vi "Main.vi"(10 "MCP Sub Panel":refnum<vi>, 11 "Module Admin":refnum<class "Delacor_lib_QMH_Module Admin.lvclass">) -> ()   [LabVIEW 2020, in "Money Control Pane.lvlib"]
doc: "This template is based off of the Queued Message Handler design pattern and the Queued Message Handler project template that ships with LabVIEW.\n\nThe main difference is that the queue is private to this module and communication between modules is performed via Broadcast and Request events.\n\nRequest events are wrapped in public API methods and are handled in the Event Handling Loop (EHL) of this VI. Any module can register for Broadcast events sent by this module. The EHL generates messages based on user interface actions.\n\nThe Message Handling Loop (MHL) processes messages generated by the EHL, or by other messages. The messages are string values, so new messages can be added easily to the Message Cases case structure in the MHL. Each message cluster can also provide an optional value for Message Data, which is a variant that can be converted to whatever message-specific data is required.\n_____\nBased on Delacor QMH Project Template 5.0.0.82."
uses:
  Money Control Pane.lvlib
  <vilib>/Delacor/Delacor QMH/Libraries/Module Admin_class/Delacor_lib_QMH_Module Admin.lvclass
  Module Data--cluster.ctl
  Stop Argument--cluster.ctl
  <vilib>/Delacor/Delacor QMH/Libraries/Message Queue_class/Delacor_lib_QMH_Message Queue.lvclass/Delacor_lib_QMH_Message Queue.ctl
  <vilib>/Delacor/Delacor QMH/Libraries/Module Admin_class/Delacor_lib_QMH_Module Admin.lvclass/Delacor_lib_QMH_Module Admin.ctl
  Configuration Change Argument--cluster.ctl
  TypeDefinitions/CurrencyEnum.ctl
  <vilib>/Utility/miscctls.llb/LVPointTypeDef.ctl
  <vilib>/Delacor/Delacor QMH/Libraries/Message Queue_class/Delacor_lib_QMH_Enqueue Message (Single).vi
  <vilib>/Delacor/Delacor QMH/Libraries/Module Admin_class/Delacor_lib_QMH_Get External Launch.vi
  <vilib>/Utility/error.llb/Error Cluster From Error Code.vi
  <vilib>/ErrorRing/Error Ring.xnode
  <vilib>/Delacor/Delacor QMH/Libraries/Message Queue_class/Delacor_lib_QMH_Message Queue.lvclass
  Config Files Management/Config File Management.lvlib
panel:
  out "value":dbl
  in  "Coins":T1
  out "error out":errorcluster
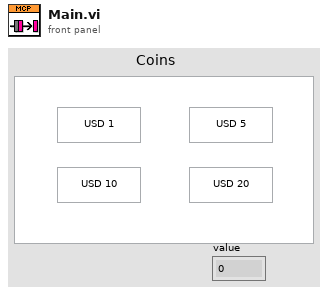
[diagram p1: front panel]
types:
  T1 = cluster{"Coin 1":bool, "Coin 2":bool, "Coin 3":bool, "Coin 4":bool}
  T2 = typedef "Money Control Pane.lvlib/Request Events--cluster.ctl" = cluster{"Stop Module":refnum<user-event>, "Show Panel":refnum<user-event>, "Hide Panel":refnum<user-event>, "Get Module Execution Status":refnum<user-event>, "Show Diagram":refnum<user-event>, "Configuration Change":refnum<user-event>}
  T3 = typedef "Money Control Pane.lvlib/Module Data--cluster.ctl" = cluster{"Status":string, "Coin Array":string[], "Values":dbl[]}
  T4 = enum32{"invalid lock state", "Not Locked", "Locked (No Password)", "Password-protected"}
  T5 = typedef "Money Control Pane.lvlib/Stop Argument--cluster.ctl" = cluster{"Origin":string, "Exit via Stop Module Req?":bool, "Wait for Module to stop?":bool}
  T6 = typedef "Money Control Pane.lvlib/Configuration Change Argument--cluster.ctl" = cluster{"Enum":T7}
  T7 = typedef "CurrencyEnum.ctl" = enum16{"USD", "MXN", "EUR", "GBP"}
  T8 = typedef "LVPointTypeDef.ctl" = cluster{"Horizontal":i16, "Vertical":i16}
  T9 = enum32{"Invalid", "Standard", "Closed", "Hidden", "Minimized", "Maximized"}
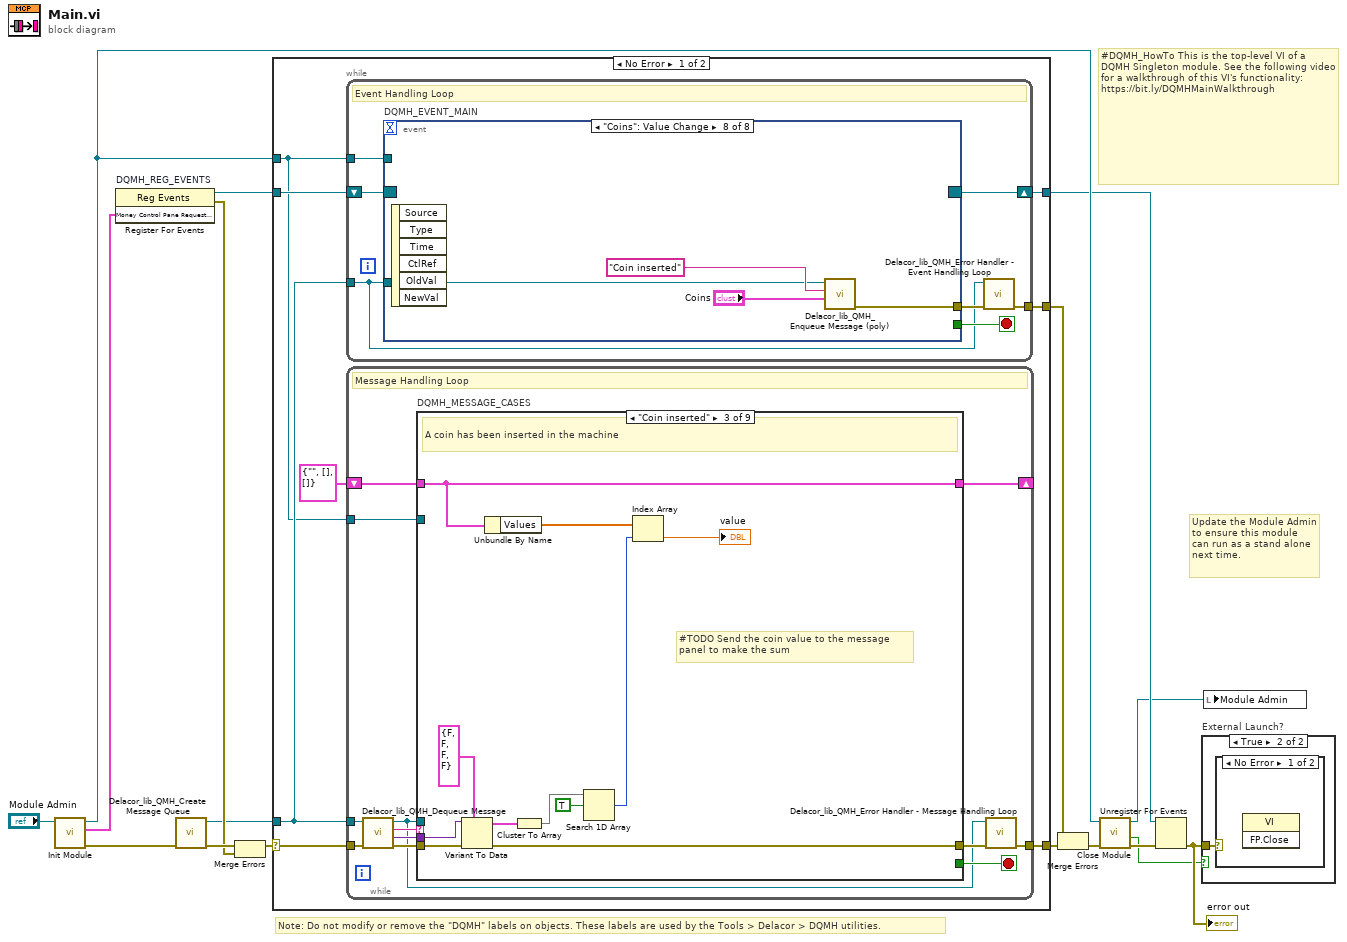
[diagram p0: block diagram]
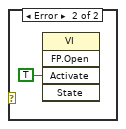
[diagram p3: hidden frame]
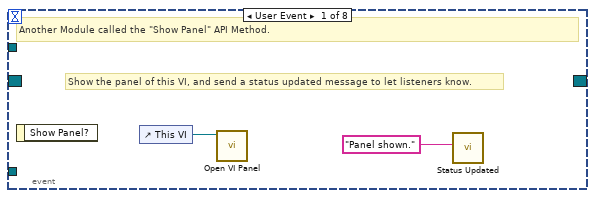
[diagram p4: hidden frame]
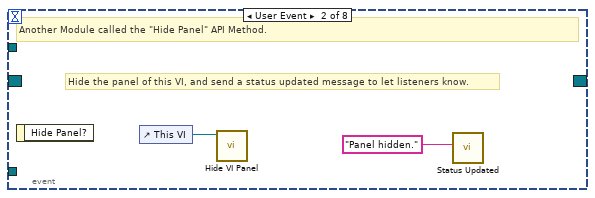
[diagram p5: hidden frame]
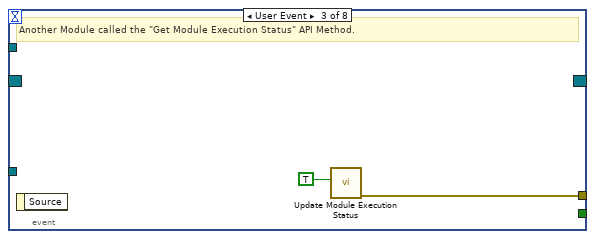
[diagram p6: hidden frame]
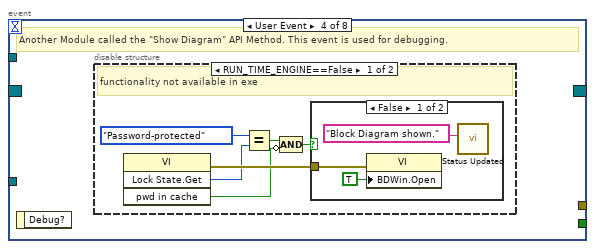
[diagram p7: hidden frame]
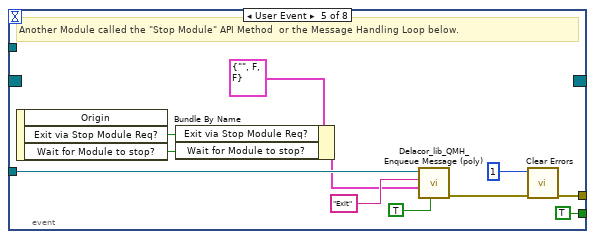
[diagram p10: hidden frame]
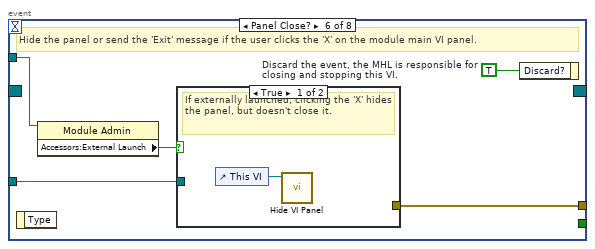
[diagram p11: hidden frame]
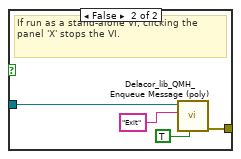
[diagram p12: hidden frame]
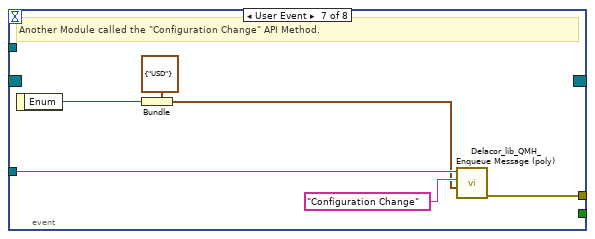
[diagram p13: hidden frame]
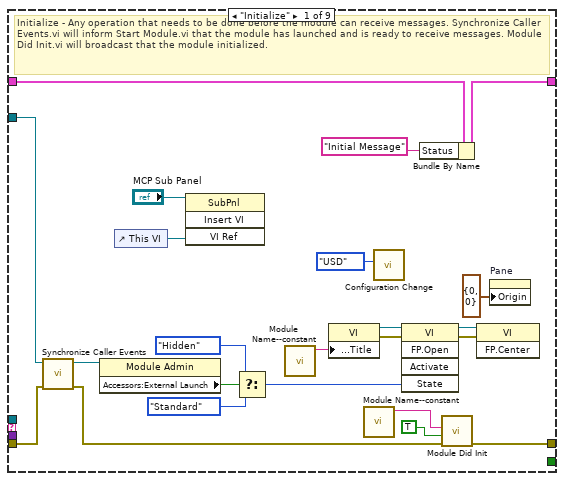
[diagram p14: hidden frame]
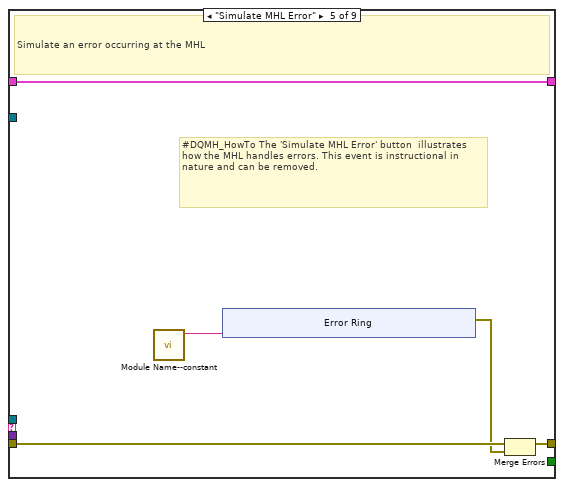
[diagram p17: hidden frame]
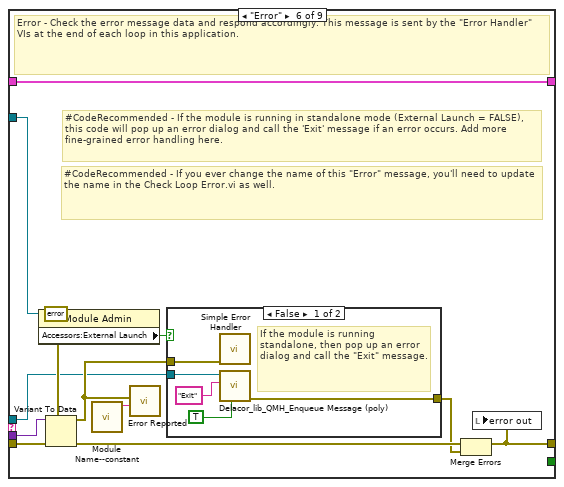
[diagram p18: hidden frame]
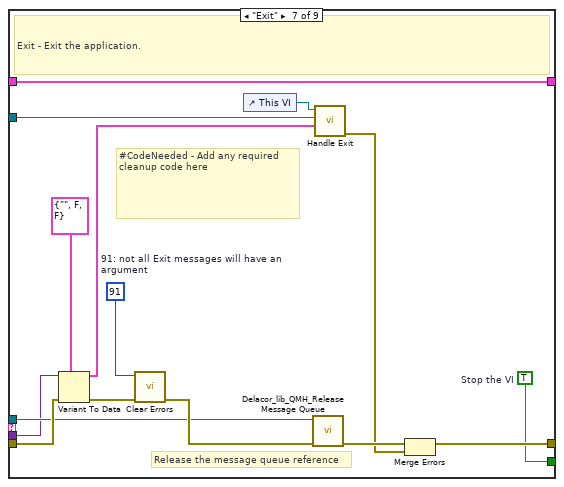
[diagram p20: hidden frame]
diagram:
  # "#DQMH_HowTo This is the top-level VI of a DQMH Singleton module. See the following video for a walkthrough of this VI's functionality: https://bit.ly/DQMHMainWalkthrough"
  # "Note: Do not modify or remove the \"DQMH\" labels on objects. These labels are used by the Tools > Delacor > DQMH utilities."
  # "Update the Module Admin to ensure this module can run as a stand alone next time."
  n1 = call "Init Module.vi"("Singleton Module Admin in"="Module Admin") -> ("error out"=w16:errorcluster, "Money Control Pane Request Events"=w5:T2, "Singleton Module Admin out"=w8:refnum<class "Delacor_lib_QMH_Module Admin.lvclass">)  [unwired: 8 in]
  n2 = register-events "DQMH_REG_EVENTS"(w5) -> (reference out=w6:refnum<event-registration>, error out=w9:errorcluster)  [unwired: 2 in]
  n3 = call <vilib>:"Delacor_lib_QMH_Create Message Queue.vi"("error in (no error)"=w16) -> ("error out"=w11:errorcluster, "Message Queue"=w4:refnum<class "Delacor_lib_QMH_Message Queue.lvclass">)  [unwired: 9 in]
  n4 = Merge Errors(w11, w9) -> (w10:errorcluster)
  n5 = case shown="No Error" w10 {
    selector: w10 -> [w23 w204]
    tunnel: [w25 w203] -> w17
    tunnel: [w22 w209] -> w7
    tunnel: w6 -> [w20 w209]
    tunnel: w4 -> [w19 w202]
    tunnel: [w24 _] -> w14
    tunnel: w8 -> [w18 w205]
    frame No Error {
      n6 = while {
        tunnel: w19 -> [w26]
        shift-right: [w29] -> w22
        shift-left: w20 -> [w30]
        tunnel: [w31] -> w24
        tunnel: w18 -> [w27]
        stop <- w28 stop-if-true
        # "Event Handling Loop"
        n7 = event "DQMH_EVENT_MAIN" shown="[7] \"Coins\": Value Change" {
          selector: w30 -> [_ _ _ _ _ _ _ _]
          dyn-events: [_ _ _ _ _ _ _ _] -> w29
          timeout: _ -> [_ _ _ _ _ _ _ _]
          tunnel: [_ _ _ _ TRUE ("Discard?") _ _ _] -> w28
          tunnel: w26 -> [_ _ _ _ w54 w61 w74 w77]
          tunnel: [_ _ w38 _ w57 w63 w69 w76] -> w32
          tunnel: w27 -> [_ _ _ _ _ w60 _ _]
          event User Event {
            # "Show the panel of this VI, and send a status updated message to let listeners know."
            # "Another Module called the \"Show Panel\" API Method."
            n8 = event-data() -> ()  [unwired: 1 in, 1 out]
            n9 = control-ref of="This VI"() -> (w34:refnum<vi>)
            n10 = call "Open VI Panel.vi"("VI"=w34) -> ()  [unwired: 10 in, 1 out]
            n11 = call "Status Updated.vi"("Status"="Panel shown." ("format string")) -> ()  [unwired: 10 in, 1 out]
          }
          event User Event {
            # "Hide the panel of this VI, and send a status updated message to let listeners know."
            # "Another Module called the \"Hide Panel\" API Method."
            n12 = event-data() -> ()  [unwired: 1 in, 1 out]
            n13 = control-ref of="This VI"() -> (w36:refnum<vi>)
            n14 = call "Hide VI Panel.vi"("VI"=w36) -> ()  [unwired: 10 in, 1 out]
            n15 = call "Status Updated.vi"("Status"="Panel hidden." ("format string")) -> ()  [unwired: 10 in, 1 out]
          }
          event User Event {
            # "Another Module called the \"Get Module Execution Status\" API Method."
            n16 = event-data() -> ()  [unwired: 1 in, 1 out]
            n17 = call "Update Module Execution Status.vi"("Running?"=TRUE) -> ("error out"=w38:errorcluster)  [unwired: 10 in]
          }
          event User Event {
            # "Another Module called the \"Show Diagram\" API Method. This event is used for debugging."
            n18 = event-data() -> ()  [unwired: 1 in, 1 out]
            n19 = disable-structure shown="RUN_TIME_ENGINE==False" {
              frame condition #0 (active) {
                # "functionality not available in exe"
                n20 = invoke class="VI" method="Lock State.Get"() -> (error out=w44:errorcluster, "Get Lock State"=w43:T4, "pwd in cache"=w40:bool)  [unwired: 4 in, 1 out]
                n21 = Equal?(x=T4."Password-protected", y=w43) -> (x = y?=w41:bool)
                n22 = Compound Arithmetic op=AND(w41, invert w40) -> (w39:bool)
                n23 = case shown="False" w39 {
                  tunnel: w44 -> [w47 _]
                  frame False {
                    n24 = property class="VI"(error in=w47, "BDWin.Open"=TRUE ("Block Diagram Window:Open")) -> ()  [unwired: 1 in, 2 out]
                    n25 = call "Status Updated.vi"("Status"="Block Diagram shown." ("format string")) -> ()  [unwired: 10 in, 1 out]
                  }
                  frame True {
                    # "Password-protected VI, and the password is not in the cache. Do not show the diagram."
                  }
                }
              }
              frame condition #1 {
              }
            }
          }
          event User Event {
            # "Another Module called the \"Stop Module\" API Method  or the Message Handling Loop below."
            n26 = event-data() -> ("Exit via Stop Module Req?"=w50:bool, "Wait for Module to stop?"=w49:bool)  [unwired: 1 in, 1 out]
            n27 = Bundle By Name(cluster=T5 {"Origin"="", "Exit via Stop Module Req?"=FALSE, "Wait for Module to stop?"=FALSE} ("Stop Argument"), "Exit via Stop Module Req?"=w50, "Wait for Module to stop?"=w49) -> (w48:T5)
            n28 = call-poly <vilib>:"Delacor_lib_QMH_Enqueue Message (poly).vi"("Priority Message? (F)"=TRUE, "Message Data"=w48, "Message"="Exit", "Message Queue in"=w54) -> ("error out"=w58:errorcluster)  [unwired: 6 in, 1 out]
            n29 = call <vilib>:"Clear Errors.vi"("error in (no error)"=w58, "specific error code to clear (0: all)"=1) -> ("error out"=w57:errorcluster)  [unwired: 4 in, 1 out]
          }
          event Panel Close? {
            w62 = TRUE  # Discard the event, the MHL is responsible for closing and stopping this VI.
            # "Hide the panel or send the 'Exit' message if the user clicks the 'X' on the module main VI panel."
            n30 = event-data() -> ()  [unwired: 1 in, 1 out]
            n31 = property class="Module Admin"(reference=w60) -> ("Accessors:External Launch"=w59:bool)  [unwired: 1 in, 2 out]
            n32 = case shown="True" w59 {
              tunnel: w61 -> [_ w67]
              tunnel: [_ w68] -> w63
              frame True {
                # "If externally launched, clicking the 'X' hides the panel, but doesn't close it."
                n33 = control-ref of="This VI"() -> (w64:refnum<vi>)
                n34 = call "Hide VI Panel.vi"("VI"=w64) -> ()  [unwired: 10 in, 1 out]
              }
              frame False {
                # "If run as a stand-alone VI, clicking the panel 'X' stops the VI."
                n35 = call-poly <vilib>:"Delacor_lib_QMH_Enqueue Message (poly).vi"("Priority Message? (F)"=TRUE, "Message"="Exit", "Message Queue in"=w67) -> ("error out"=w68:errorcluster)  [unwired: 7 in, 1 out]
              }
            }
            n36 = event-data("Discard?"=w62) -> ()  [unwired: 1 in, 1 out]
          }
          event User Event {
            # "Another Module called the \"Configuration Change\" API Method."
            n37 = event-data() -> ("Enum"=w70:T7)  [unwired: 1 in]
            n38 = Bundle(cluster=T6 {"Enum"=enum."USD"} ("Configuration Change Argument"), "Enum"=w70) -> (w71:T6)
            n39 = call-poly <vilib>:"Delacor_lib_QMH_Enqueue Message (poly).vi"("Message Data"=w71, "Message"="Configuration Change", "Message Queue in"=w74) -> ("error out"=w69:errorcluster)  [unwired: 7 in, 1 out]
          }
          event "Coins": Value Change {
            n40 = event-data() -> ()  [unwired: 1 in, 6 out]
            n41 = call-poly <vilib>:"Delacor_lib_QMH_Enqueue Message (poly).vi"("Message Data"="Coins", "Message"="Coin inserted", "Message Queue in"=w77) -> ("error out"=w76:errorcluster)  [unwired: 7 in, 1 out]
          }
        }
        n42 = call-dynamic "Delacor_lib_QMH_Error Handler - Event Handling Loop.vi"("error in (no error)"=w32, "Message Queue in"=w26) -> ("dup error in"=w31:errorcluster)  [unwired: 8 in, 1 out]
      }
      n43 = while {
        tunnel: w19 -> [w81]
        shift-right: [w85] -> _
        shift-left: T3 {"Status"="", "Coin Array"=[], "Values"=[]} ("Data Cluster") -> [w86]
        tunnel: w23 -> [w89]
        tunnel: [w87] -> w25
        tunnel: w18 -> [w79]
        stop <- w84 stop-if-true
        # "Message Handling Loop"
        n44 = call-dynamic "Delacor_lib_QMH_Dequeue Message.vi"("error in (no error)"=w89, "Message Queue in"=w81) -> ("error out"=w88:errorcluster, "Message Data"=w82:variant, "Message"=w83:string, "Message Queue out"=w80:refnum<class "Delacor_lib_QMH_Message Queue.lvclass">)  [unwired: 6 in]
        n45 = case "DQMH_MESSAGE_CASES" shown="\"Coin inserted\"" w83 {
          selector: w83 -> [_ _ _ _ _ _ _ w174 _]
          tunnel: w80 -> [_ _ _ _ _ w144 w166 _ _]
          tunnel: w88 -> [w111 w115 w126 w128 w133 w151 w172 w176 w201]
          tunnel: [w109 w115 w125 w128 w132 w147 w169 w177 w188] -> w90
          tunnel: w86 -> [w100 w114 w119 w127 w130 w146 w165 w175 w200]
          tunnel: [w99 w114 w119 w127 w130 w146 w165 w175 w191] -> w85
          tunnel: [_ _ _ _ _ _ w164 _ _] -> w84
          tunnel: w82 -> [_ _ w124 _ _ w145 w163 _ w198]
          tunnel: w79 -> [w101 _ _ _ _ w143 w158 _ _]
          frame "Initialize" {
            # "Initialize - Any operation that needs to be done before the module can receive messages. Synchronize Caller Events.vi will inform Start Module.vi that the module has launched and is ready to receive messages. Module Did Init.vi will broadcast that the module initialized."
            n46 = call "Synchronize Caller Events.vi"("error in (no error)"=w111, "Singleton Module Admin in"=w101) -> ("error out"=w110:errorcluster, "Singleton Module Admin out"=w96:refnum<class "Delacor_lib_QMH_Module Admin.lvclass">)  [unwired: 8 in]
            n47 = property class="Module Admin"(reference=w96) -> ("Accessors:External Launch"=w105:bool)  [unwired: 1 in, 2 out]
            n48 = control-ref of="This VI"() -> (w92:refnum<vi>)
            n49 = invoke class="SubPnl" method="Insert VI"(reference="MCP Sub Panel", "VI Ref"=w92) -> ()  [unwired: 2 in, 4 out]
            n50 = Select(t=T9."Hidden" ("State"), s=w105, f=T9."Standard" ("State")) -> (s? t:f=w102:T9)
            n51 = call "Module Name--constant.vi"() -> ("Module Name"=w108:string)  [unwired: 11 in]
            n52 = property class="VI"("Front Panel.Title"=w108) -> (reference out=w107:refnum<vi>, error out=w113:errorcluster)  [unwired: 2 in]
            n53 = call "Module Name--constant.vi"() -> ("Module Name"=w97:string)  [unwired: 11 in]
            n54 = call "Configuration Change.vi"("Enum"=CurrencyEnum."USD") -> ()  [unwired: 10 in, 1 out]
            n55 = invoke class="VI" method="FP.Open"(reference=w107, error in=w113, "State"=w102) -> (reference out=w106:refnum<vi>, error out=w112:errorcluster)  [unwired: 2 in, 3 out]
            n56 = Bundle By Name(cluster=w100, "Status"="Initial Message" ("Initial Message")) -> (w99:T3)
            n57 = call "Module Did Init.vi"("error in (no error)"=w110, "Initialized?"=TRUE, "Origin"=w97) -> ("error out"=w109:errorcluster)  [unwired: 8 in]
            n58 = invoke class="VI" method="FP.Center"(reference=w106, error in=w112) -> ()  [unwired: 1 in, 3 out]
            n59 = property on="Pane" class="Pane"("Origin"=T8 {"Horizontal"=0, "Vertical"=0}) -> ()  [unwired: 2 in, 2 out]
          }
          frame "--- Module Specific ---" {
            # "Separator -- The following cases handle messages specific to this Module."
          }
          frame "Coin inserted" {
            # "#TODO Send the coin value to the message \npanel to make the sum"
            # "A coin has been inserted in the machine"
            n60 = Variant To Data(error in=w126, type=T1 {"Coin 1"=FALSE, "Coin 2"=FALSE, "Coin 3"=FALSE, "Coin 4"=FALSE} ("Coins"), Variant=w124) -> (data=w122:T1, error out=w125:errorcluster)
            n61 = Unbundle By Name(w119) -> ("Values"=w118:dbl[])
            n62 = Cluster To Array(cluster=w122) -> (array=w121:bool[])
            n63 = Search 1D Array(1D array=w121, element=TRUE) -> (index of element=w117:i32)  [unwired: 1 in]
            n64 = Index Array(array=w118, index=w117) -> (element=→"value":dbl)
          }
          frame "--- Exit and Error Handling---" {
            # "Separator - The following cases handle errors and exit messages."
          }
          frame "Simulate MHL Error" {
            # "#DQMH_HowTo The 'Simulate MHL Error' button  illustrates how the MHL handles errors. This event is instructional in nature and can be removed."
            # "Simulate an error occurring at the MHL"
            n65 = call "Module Name--constant.vi"() -> ("Module Name"=w129:string)  [unwired: 11 in]
            n66 = xnode "Error Ring"("parameter 0"=w129) -> ("error out"=w131:errorcluster)
            n67 = Merge Errors(w133, w131) -> (w132:errorcluster)
          }
          frame "Error" {
            # "#CodeRecommended - If you ever change the name of this \"Error\" message, you'll need to update the name in the Check Loop Error.vi as well."
            # "#CodeRecommended - If the module is running in standalone mode (External Launch = FALSE), this code will pop up an error dialog and call the 'Exit' message if an error occurs. Add more fine-grained error handling here."
            # "Error - Check the error message data and respond accordingly. This message is sent by the \"Error Handler\" VIs at the end of each loop in this application."
            n68 = property class="Module Admin"(reference=w143) -> ("Accessors:External Launch"=w142:bool)  [unwired: 1 in, 2 out]
            n69 = Variant To Data(error in=w151, type=errorcluster {"status"=FALSE, "code"=0, "source"=""} ("error constant"), Variant=w145) -> (data=w152:errorcluster, error out=w149:errorcluster)
            n70 = call "Module Name--constant.vi"() -> ("Module Name"=w141:string)  [unwired: 11 in]
            n71 = call "Error Reported.vi"("Additional Information"=w141, "Error"=w152) -> ()  [unwired: 9 in, 1 out]
            n72 = case shown="False" w142 {
              tunnel: [w157 _] -> w148
              tunnel: w144 -> [w155 _]
              tunnel: w152 -> [w156 _]
              frame False {
                # "If the module is running standalone, then pop up an error dialog and call the \"Exit\" message."
                n73 = call <vilib>:"Simple Error Handler.vi"("error in (no error)"=w156) -> ()  [unwired: 4 in, 5 out]
                n74 = call-poly <vilib>:"Delacor_lib_QMH_Enqueue Message (poly).vi"("Priority Message? (F)"=TRUE, "Message"="Exit", "Message Queue in"=w155) -> ("error out"=w157:errorcluster)  [unwired: 7 in, 1 out]
              }
              frame True {
                # "If the module was launched externally, calling the Error Reported broadcast VI is the only action performed by the \"Error\" message. The module's caller can then process the error appropriately."
              }
            }
            n75 = Merge Errors(w149, w148) -> (w147:errorcluster)
            n76 = local write "error out"(w147) -> ()
          }
          frame "Exit" {
            w162 = 91  # 91: not all Exit messages will have an argument
            w164 = TRUE  # Stop the VI
            # "Release the message queue reference"
            # "#CodeNeeded - Add any required cleanup code here"
            # "Exit - Exit the application."
            n77 = Variant To Data(error in=w172, type=T5 {"Origin"="", "Exit via Stop Module Req?"=FALSE, "Wait for Module to stop?"=FALSE} ("Stop Argument"), Variant=w163) -> (data=w160:T5, error out=w168:errorcluster)
            n78 = call <vilib>:"Clear Errors.vi"("error in (no error)"=w168, "specific error code to clear (0: all)"=w162) -> ("error out"=w171:errorcluster)  [unwired: 4 in, 1 out]
            n79 = control-ref of="This VI"() -> (w159:refnum<vi>)
            n80 = call-dynamic "Delacor_lib_QMH_Release Message Queue.vi"("error in (no error)"=w171, "Message Queue"=w166) -> ("error out"=w170:errorcluster)  [unwired: 9 in]
            n81 = call "Handle Exit.vi"("Stop Argument"=w160, "Admin in"=w158, "VI reference"=w159) -> ("error out"=w167:errorcluster)  [unwired: 7 in, 1 out]
            n82 = Merge Errors(w170, w167) -> (w169:errorcluster)
          }
          frame Default {
            # "'Default' case only runs if there is a message that isn't defined in any of the other cases.  Output a programming error."
            n83 = call "Module Name--constant.vi"() -> ("Module Name"=w173:string)  [unwired: 11 in]
            n84 = xnode "Error Ring"("parameter 0"=w174, "parameter 1"=w173) -> ("error out"=w178:errorcluster)
            n85 = Merge Errors(w176, w178) -> (w177:errorcluster)
          }
          frame "Configuration Change" {
            # "Sets a configuration change done by the settings window or the VI itself."
            n86 = Variant To Data(error in=w201, type=T6 {"Enum"=enum."USD"} ("Configuration Change Argument"), Variant=w198) -> (error out=w199:errorcluster)  [unwired: 1 out]
            n87 = call "Create Currency Map.vi"() -> ("error out"=w187:errorcluster, "Value"=w190:dbl[], "Denomination"=w189:string[])  [unwired: 9 in]
            n88 = control-ref of="Coin 1"() -> (w195:refnum<vi>)
            n89 = control-ref of="Coin 2"() -> (w194:refnum<vi>)
            n90 = control-ref of="Coin 3"() -> (w193:refnum<vi>)
            n91 = control-ref of="Coin 4"() -> (w192:refnum<vi>)
            n92 = Build Array(w195, w194, w193, w192) -> (w196:refnum<vi>[])
            n93 = call "Write Values on Buttons.vi"("Coin Array"=w189, "appended array"=w196) -> ()  [unwired: 10 in]
            n94 = Bundle By Name(cluster=w200, "Coin Array"=w189, "Values"=w190) -> (w191:T3)
            n95 = Merge Errors(w187, w199) -> (w188:errorcluster)
          }
        }
        n96 = call-dynamic "Delacor_lib_QMH_Error Handler - Message Handling Loop.vi"("error in (no error)"=w90, "Message Queue in"=w80) -> ("dup error in"=w87:errorcluster)  [unwired: 8 in, 1 out]
      }
    }
    frame Error {
      # "Synchronize Caller Events.vi will inform Start Module.vi that the module has launched and will let the code calling Start Module.vi register for broadcasts and would permit the caller receive the broadcast that an error occurred at launch time."
      n97 = call-dynamic "Delacor_lib_QMH_Release Message Queue.vi"("error in (no error)"=w204, "Message Queue"=w202) -> ("error out"=w203:errorcluster)  [unwired: 9 in]
      n98 = call "Synchronize Caller Events.vi"("Singleton Module Admin in"=w205) -> ("error out"=w210:errorcluster)  [unwired: 9 in, 1 out]
      n99 = call "Module Name--constant.vi"() -> ("Module Name"=w208:string)  [unwired: 11 in]
      n100 = Format Into String(format string="An error occurred during initialization. %s is no longer running.", w208) -> (resulting string=w206:string)  [unwired: 2 in, 1 out]
      n101 = Merge Errors(w203, w210) -> (w211:errorcluster)
      n102 = call "Error Reported.vi"("Additional Information"=w206, "Error"=w211) -> ()  [unwired: 9 in, 1 out]
    }
  }
  n103 = Merge Errors(w14, w17) -> (w13:errorcluster)
  n104 = call "Close Module.vi"("error in (no error)"=w13, "Module Admin in"=w8) -> ("error out"=w15:errorcluster, "External Launch"=w1:bool, "Module Admin out"=w2:refnum<class "Delacor_lib_QMH_Module Admin.lvclass">)  [unwired: 7 in]
  n105 = Unregister For Events(event registration refnum=w7, error in=w15) -> (error out=w12:errorcluster)
  "error out" <- w12
  n106 = case "External Launch?" shown="True" w1 {
    tunnel: w12 -> [_ w212]
    frame False {
    }
    frame True {
      n107 = case shown="No Error" w212 {
        frame No Error {
          n108 = invoke class="VI" method="FP.Close"() -> ()  [unwired: 3 in, 3 out]
        }
        frame Error {
          n109 = invoke class="VI" method="FP.Open"("Activate"=TRUE ("Activate?")) -> ()  [unwired: 4 in, 5 out]
        }
      }
    }
  }
  n110 = local write "Module Admin"(w2) -> ()
